vi "CREATE SUB CALIBRATION DATA.vi"(11 "Calibration Factor":T1) -> (3 "OUT":dbl[](array[numeric]))   [LabVIEW 2015]
uses:
  Calibration/calibration.ctl
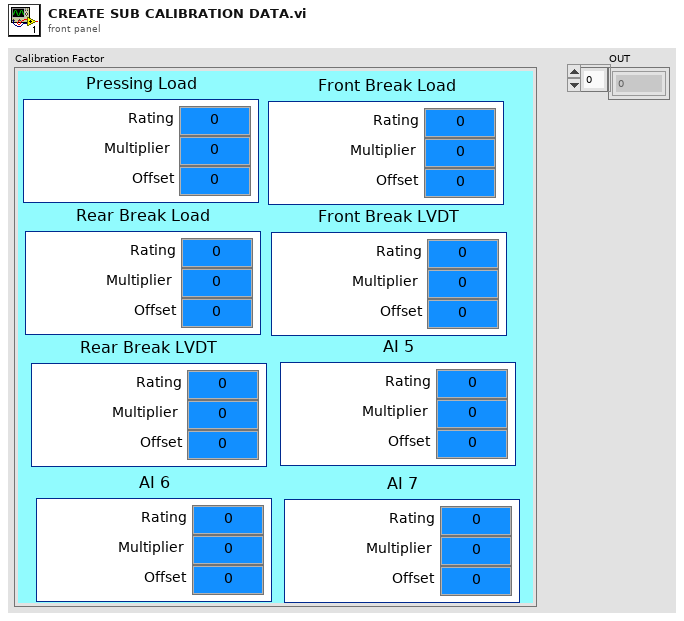
[diagram p1: front panel]
types:
  T1 = typedef "calibration.ctl" = cluster{"Pressing Load":cluster{"Rating":dbl, "Multiplier":dbl, "Offset":dbl}, "Front Break Load":cluster{"Rating":dbl, "Multiplier":dbl, "Offset":dbl}, "Rear Break Load":cluster{"Rating":dbl, "Multiplier":dbl, "Offset":dbl}, "Front Break LVDT":cluster{"Rating":dbl, "Multiplier":dbl, "Offset":dbl}, "Rear Break LVDT":cluster{"Rating":dbl, "Multiplier":dbl, "Offset":dbl}, "AI 5":cluster{"Rating":dbl, "Multiplier":dbl, "Offset":dbl}, "AI 6":cluster{"Rating":dbl, "Multiplier":dbl, "Offset":dbl}, "AI 7":cluster{"Rating":dbl, "Multiplier":dbl, "Offset":dbl}}
  T2 = cluster{"Rating":dbl, "Multiplier":dbl, "Offset":dbl}
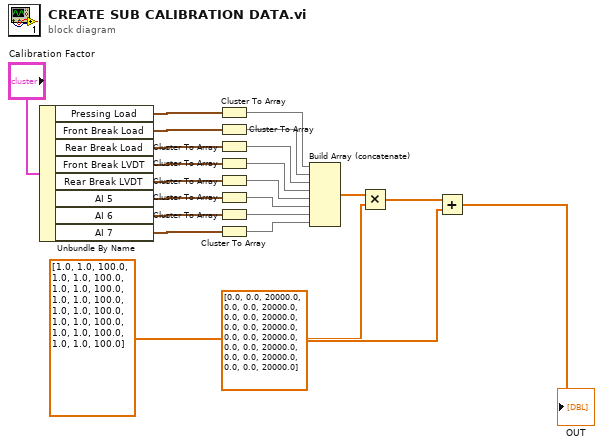
[diagram p0: block diagram]
diagram:
  n1 = Unbundle By Name("Calibration Factor") -> ("Pressing Load"=w1:T2, "Front Break Load"=w2:T2, "Rear Break Load"=w3:T2, "Front Break LVDT"=w4:T2, "Rear Break LVDT"=w8:T2, "AI 5"=w7:T2, "AI 6"=w6:T2, "AI 7"=w5:T2)
  n2 = Cluster To Array(cluster=w1) -> (array=w9:dbl[])
  n3 = Cluster To Array(cluster=w2) -> (array=w10:dbl[])
  n4 = Cluster To Array(cluster=w3) -> (array=w11:dbl[])
  n5 = Cluster To Array(cluster=w4) -> (array=w12:dbl[])
  n6 = Cluster To Array(cluster=w8) -> (array=w13:dbl[])
  n7 = Cluster To Array(cluster=w7) -> (array=w14:dbl[])
  n8 = Cluster To Array(cluster=w6) -> (array=w15:dbl[])
  n9 = Cluster To Array(cluster=w5) -> (array=w16:dbl[])
  n10 = Build Array (concatenate)(w9, w10, w11, w12, w13, w14, w15, w16) -> (w17:dbl[])
  n11 = Multiply(x=w17, y=dbl[] [1.0, 1.0, 100.0, 1.0, 1.0, 100.0, 1.0, 1.0, 100.0, 1.0, 1.0, 100.0, 1.0, 1.0, 100.0, 1.0, 1.0, 100.0, 1.0, 1.0, 100.0, 1.0, 1.0, 100.0] ("initialized array")) -> (x*y=w20:dbl[])
  n12 = Add(x=w20, y=dbl[] [0.0, 0.0, 20000.0, 0.0, 0.0, 20000.0, 0.0, 0.0, 20000.0, 0.0, 0.0, 20000.0, 0.0, 0.0, 20000.0, 0.0, 0.0, 20000.0, 0.0, 0.0, 20000.0, 0.0, 0.0, 20000.0] ("initialized array")) -> (x+y=→"OUT":dbl[])
